vi "Gen Run Hours Latch.vi"(3 "Gen Data In":T1={"ControllerMode"=0, "Alarm"=FALSE, "Com Fault"=TRUE, "Alarms"=[], "ActivePower"=[], "ReactivePower"=[], "RunHours"=[], "ApparentPower"=[], "FuelRate"=[], "TotalFuel"=[], "PowerFactor"=[], "Frequency"=[], "BatteryVoltage"=[], "DefLevel"=[]} {"DefLevel" format="%04x"; "BatteryVoltage" format="%04x"; "Frequency" format="%04x"; "PowerFactor" format="%04x"; "ControllerMode" format="%04x"; "TotalFuel" format="%04x"; "FuelRate" format="%04x"; "ApparentPower" format="%04x"; "RunHours" format="%04x"; "ReactivePower" format="%04x"; "ActivePower" format="%04x"; "Alarms" format="%04x"}) -> (1 "Gen Data Out":T1={"ControllerMode"=0, "Alarm"=FALSE, "Com Fault"=TRUE, "Alarms"=[], "ActivePower"=[], "ReactivePower"=[], "RunHours"=[], "ApparentPower"=[], "FuelRate"=[], "TotalFuel"=[], "PowerFactor"=[], "Frequency"=[], "BatteryVoltage"=[], "DefLevel"=[]} {"DefLevel" format="%04x"; "BatteryVoltage" format="%04x"; "Frequency" format="%04x"; "PowerFactor" format="%04x"; "ControllerMode" format="%04x"; "TotalFuel" format="%04x"; "FuelRate" format="%04x"; "ApparentPower" format="%04x"; "RunHours" format="%04x"; "ReactivePower" format="%04x"; "ActivePower" format="%04x"; "Alarms" format="%04x"})   [LabVIEW 2014]
uses:
  Controls/Gen Data.ctl
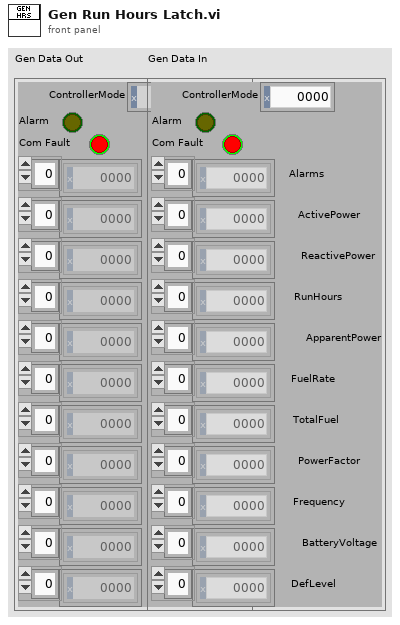
[diagram p1: front panel]
types:
  T1 = typedef "Gen Data.ctl" = cluster{"ControllerMode":u16, "Alarm":bool, "Com Fault":bool, "Alarms":u16[], "ActivePower":u16[], "ReactivePower":u16[], "RunHours":u16[], "ApparentPower":u16[], "FuelRate":u16[], "TotalFuel":u16[], "PowerFactor":u16[], "Frequency":u16[], "BatteryVoltage":u16[], "DefLevel":u16[]}
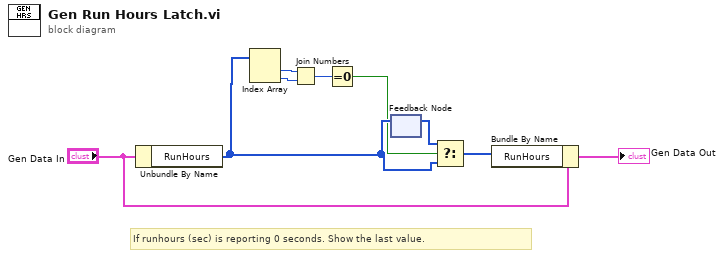
[diagram p0: block diagram]
diagram:
  # "If runhours (sec) is reporting 0 seconds. Show the last value."
  n1 = Unbundle By Name("Gen Data In") -> ("RunHours"=w5:u16[])
  n2 = Index Array(array=w5) -> (element #1=w4:u16, element #2=w3:u16)  [unwired: 2 in]
  n3 = Join Numbers(hi=w4, lo=w3) -> ((hi.lo)=w2:u32)
  n4 = Equal To 0?(x=w2) -> (x = 0?=w1:bool)
  n5 = feedback #1() -> (w6:u16[])  [unwired: 1 in]
  n6 = feedback-in #1(w5) -> ()
  n7 = Select(t=w6, s=w1, f=w5) -> (s? t:f=w9:u16[])
  n8 = Bundle By Name(cluster="Gen Data In", "RunHours"=w9) -> (→"Gen Data Out":T1)
